vi "+S2C_5190CR_Process.vi"(8 "Error In":errorcluster) -> (0 "Error Out":errorcluster)   [LabVIEW 2015]
doc: "Driver panel for the 5190CR PDU equipment."
uses:
  VIs/S2C_5190CR_Proc_Globals.vi
panel:
  out "Err":bool
  in  "Clear":bool
  out "Exit":bool
  in  "LogDepth":u32=10 caption="Log Depth"
  in  "CtrlTab":enum32{"5190CR"}(tab)
  in  "P1":T1={"P1C1"={"IP Address"="192.168.1.1", "Port"=23, "Username"="<Username>", "Password"="<Password>", "Timeout(ms)"=10000, "P1C1Exe"=FALSE}, "P1C2"={"Command"=0, "OutletPlug"=1, "Current"="", "Power"="", "Voltage"="", "Timeout(ms)"=10000, "P1C2Exe"=FALSE}, "P1C3"={"OutletPlug"=1, "OutletState"=TRUE, "PowerOnDelay(ms)"=50, "PowerOffDelay(ms)"=0, "WaitOnState"=TRUE, "Timeout(ms)"=10000, "P1C3Exe"=FALSE}} {"P1C3"."OutletPlug" items=["Outlet 1"=1, "Outlet 2"=2, "Outlet 3"=3, "Outlet 4"=4, "Outlet 5"=5, "Outlet 6"=6, "Outlet 7"=7, "Outlet 8"=8]; "P1C2"."Command" items=["Measure Current", "Measure Power", "Measure Voltage"]; "P1C2"."OutletPlug" items=["Outlet 1"=1, "Outlet 2"=2, "Outlet 3"=3, "Outlet 4"=4, "Outlet 5"=5, "Outlet 6"=6, "Outlet 7"=7, "Outlet 8"=8]}
  in  "CommLog":string caption="Communication Log"
  # "Main Cluster:\n394x886\n1 = 355x876\n2 = 355x438\n3 = 355x292\n4 = 163x438\n6 = 163x292\n8 = 163x219"
  # "PX3-5190CR Driver Panel"
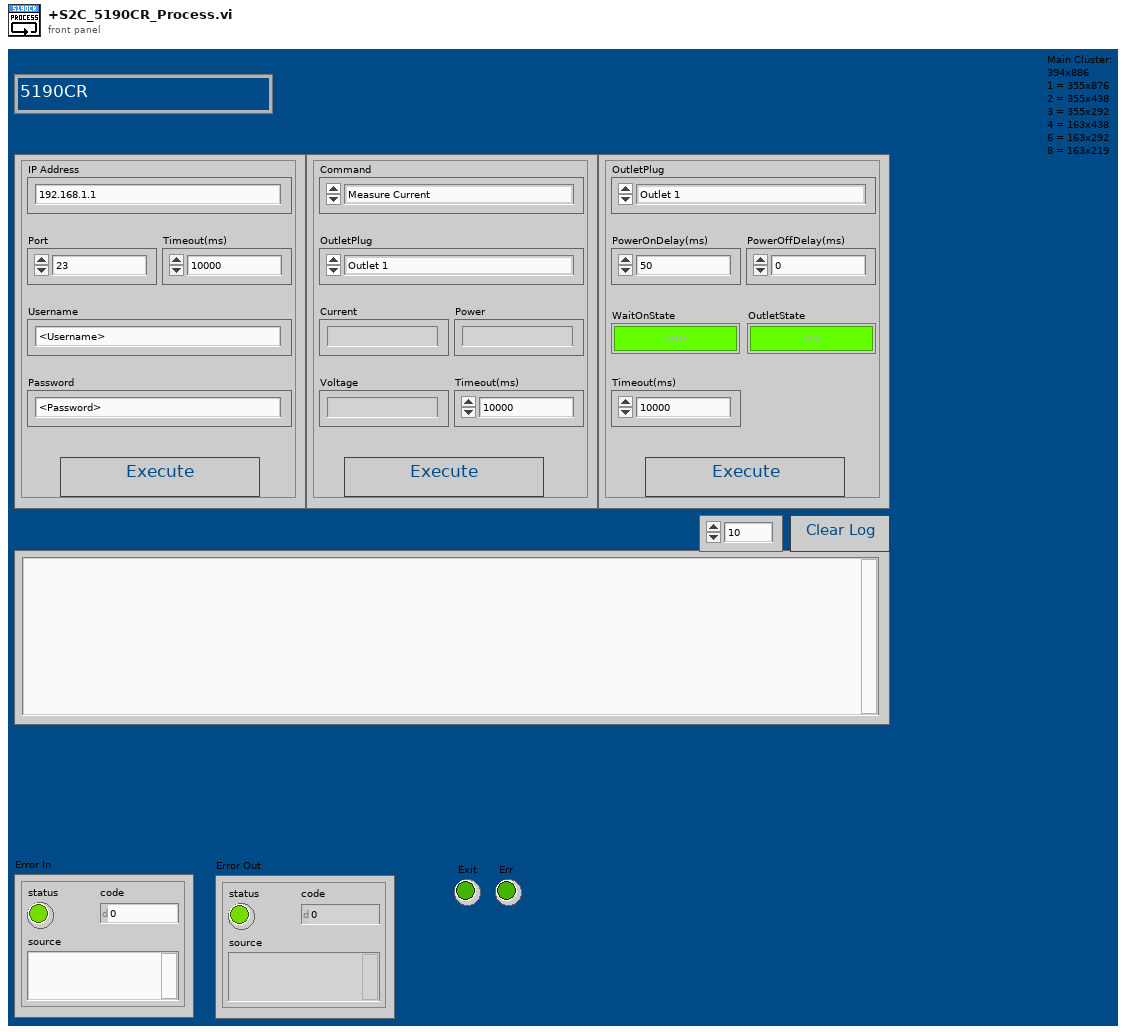
[diagram p1: front panel]
types:
  T1 = cluster{"P1C1":cluster{"IP Address":string, "Port":u16, "Username":string, "Password":string, "Timeout(ms)":i32, "P1C1Exe":bool}, "P1C2":cluster{"Command":u16, "OutletPlug":u16, "Current":string, "Power":string, "Voltage":string, "Timeout(ms)":i32, "P1C2Exe":bool}, "P1C3":cluster{"OutletPlug":u16, "OutletState":bool, "PowerOnDelay(ms)":u32, "PowerOffDelay(ms)":u32, "WaitOnState":bool, "Timeout(ms)":i32, "P1C3Exe":bool}}
  T2 = cluster{"Caller-Q":refnum<queue>, "Command":string, "Return":string, "Data":variant, "Timeout":dbl}
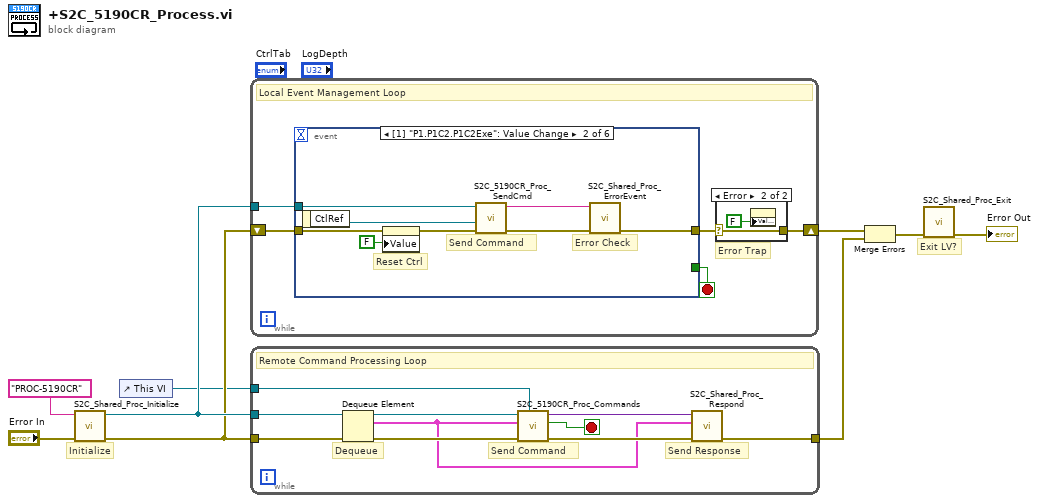
[diagram p0: block diagram]
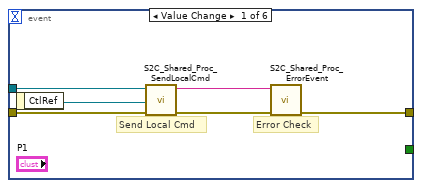
[diagram p3: hidden frame]
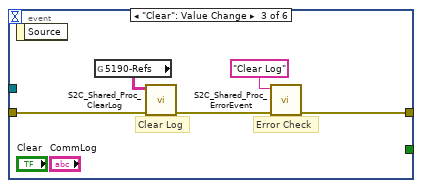
[diagram p4: hidden frame]
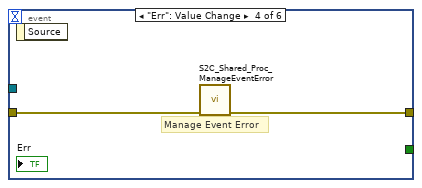
[diagram p5: hidden frame]
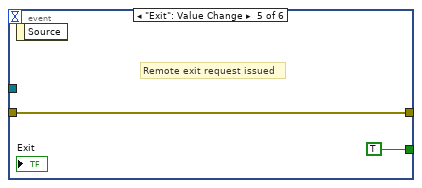
[diagram p6: hidden frame]
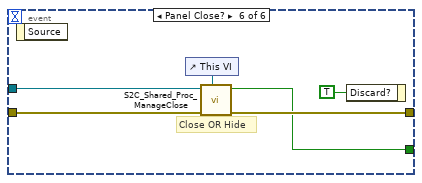
[diagram p7: hidden frame]
diagram:
  # "Exit LV?"
  # "Initialize"
  n1 = call "S2C_Shared_Proc_Initialize.vi"("Error In"="Error In", "Q-Name"="PROC-5190CR" ("name (unnamed)")) -> ("Error Out"=w4:errorcluster, "Q-Ref"=w7:refnum<queue>)  [unwired: 8 in]
  n2 = control-ref of="This VI"() -> (w1:refnum<vi>)
  n3 = while {
    tunnel: w7 -> [w13]
    shift-right: [w10] -> w6
    shift-left: w4 -> [w14]
    stop <- w12 stop-if-true
    # "Error Trap"
    # "Local Event Management Loop"
    n4 = event shown="[1] \"P1.P1C2.P1C2Exe\": Value Change" {
      selector: _ -> [_ _ _ _ _ _]
      dyn-events: _ -> [_ _ _ _ _ _]
      timeout: _ -> [_ _ _ _ _ _]
      tunnel: w14 -> [w23 w30 w36 w38 w40 w45]
      tunnel: w13 -> [w21 w31 _ _ _ w43]
      tunnel: [w19 w25 w33 w37 w40 w44] -> w11
      tunnel: [_ _ _ _ TRUE ("Discard?") w42] -> w12
      event "P1.P1C1.P1C1Exe", "P1.P1C3.P1C3Exe": Value Change {
        # "Error Check"
        # "Send Local Cmd"
        n5 = event-data() -> ("CtlRef"=w22:refnum<vi>)  [unwired: 1 in]
        n6 = call "S2C_Shared_Proc_SendLocalCmd.vi"("Error In"=w23, "ExeRef"=w22, "Q-Ref"=w21) -> ("Error Out"=w20:errorcluster, "Command"=w18:string)  [unwired: 7 in]
        n7 = call "S2C_Shared_Proc_ErrorEvent.vi"("Error In"=w20, "Command"=w18) -> ("Error Out"=w19:errorcluster)  [unwired: 9 in]
      }
      event "P1.P1C2.P1C2Exe": Value Change {
        # "Error Check"
        # "Reset Ctrl"
        # "Send Command"
        n8 = event-data() -> ("CtlRef"=w27:refnum<vi>)  [unwired: 1 in]
        n9 = property on="P1C2Exe" class="Bool (strict)"(error in=w30, "Value"=FALSE) -> (error out=w29:errorcluster)  [unwired: 1 in, 1 out]
        n10 = call "S2C_5190CR_Proc_SendCmd.vi"("Error In"=w29, "ExeRef"=w27, "Q-Ref"=w31) -> ("Error Out"=w26:errorcluster, "Command"=w24:string)  [unwired: 7 in]
        n11 = call "S2C_Shared_Proc_ErrorEvent.vi"("Error In"=w26, "Command"=w24) -> ("Error Out"=w25:errorcluster)  [unwired: 9 in]
      }
      event "Clear": Value Change {
        # "Error Check"
        # "Clear Log"
        n12 = event-data() -> ()  [unwired: 1 in, 1 out]
        n13 = global read "S2C_5190CR_Proc_Globals.vi" "5190-Refs"() -> (w35:string[][])
        n14 = call "S2C_Shared_Proc_ClearLog.vi"("Error In"=w36, "Refs"=w35) -> ("Error Out"=w34:errorcluster)  [unwired: 9 in]
        n15 = call "S2C_Shared_Proc_ErrorEvent.vi"("Error In"=w34, "Command"="Clear Log") -> ("Error Out"=w33:errorcluster)  [unwired: 9 in]
      }
      event "Err": Value Change {
        # "Manage Event Error"
        n16 = event-data() -> ()  [unwired: 1 in, 1 out]
        n17 = call "S2C_Shared_Proc_ManageEventError.vi"("Error In"=w38) -> ("Error Out"=w37:errorcluster)  [unwired: 10 in]
      }
      event "Exit": Value Change {
        # "Remote exit request issued"
        n18 = event-data() -> ()  [unwired: 1 in, 1 out]
      }
      event Panel Close? {
        # "Close OR Hide"
        n19 = event-data() -> ()  [unwired: 1 in, 1 out]
        n20 = control-ref of="This VI"() -> (w41:refnum<vi>)
        n21 = call "S2C_Shared_Proc_ManageClose.vi"("VI_Ref"=w41, "Error In"=w45, "Q-Ref"=w43) -> ("Error Out"=w44:errorcluster, "Exit?"=w42:bool)  [unwired: 7 in]
        n22 = event-data("Discard?"=TRUE) -> ()  [unwired: 1 in, 1 out]
      }
    }
    n23 = case shown="Error" w11 {
      selector: w11 -> [w15 w17]
      tunnel: [w15 w17] -> w10
      frame No Error {
      }
      frame Error {
        n24 = property on="Err" class="Bool (strict)"("Val(Sgnl)"=FALSE ("Value (Signaling)")) -> ()  [unwired: 2 in, 2 out]
      }
    }
  }
  n25 = while {
    tunnel: w7 -> [w55]
    tunnel: w1 -> [w50]
    tunnel: w4 -> [w56]
    tunnel: [w49] -> w5
    stop <- w51 stop-if-true
    # "Send Response"
    # "Send Command"
    # "Dequeue"
    # "Remote Command Processing Loop"
    n26 = Dequeue Element(queue=w55, error in (no error)=w56) -> (queue out=w48:refnum<queue>, element=w47:T2, error out=w54:errorcluster)  [unwired: 1 in, 1 out]
    n27 = call "S2C_5190CR_Proc_Commands.vi"("VI_Ref"=w50, "Error In"=w54, "Settings"=w47, "Q-Ref"=w48) -> ("Error Out"=w52:errorcluster, "Stop?"=w51:bool, "Response"=w53:variant)  [unwired: 5 in]
    n28 = call "S2C_Shared_Proc_Respond.vi"("Error In"=w52, "Settings"=w47, "Response"=w53) -> ("Error Out"=w49:errorcluster)  [unwired: 8 in]
  }
  n29 = Merge Errors(w6, w5) -> (w3:errorcluster)
  n30 = call "S2C_Shared_Proc_Exit.vi"("Error In"=w3) -> ("Error Out"=→"Error Out":errorcluster)  [unwired: 10 in]
